vi "Make Connections (Parallel).vi"(8 "error in (no error)":errorcluster, 10 "switchActionsArray":T1 {"RelayAction" items=["CloseRelay"=21, "OpenRelay"=20]}, 11 "SLSC Switch in":refnum<class "SLSC Switch.lvclass">) -> (0 "error out":errorcluster, 3 "SLSC Switch out":refnum<class "SLSC Switch.lvclass">)   [LabVIEW 2015, in "SLSC Switch.lvclass"]
uses:
  SLSC Switch.lvclass
  slscsl/SwitchActionsArray.ctl
  slscsl/SwitchAction.ctl
  slscsl/RelayAction.ctl
  SLSC Switch.lvclass/SLSC Switch.ctl
  Relay Interface/RelayInterface.lvclass
  slscsl/slscsl.lvclass
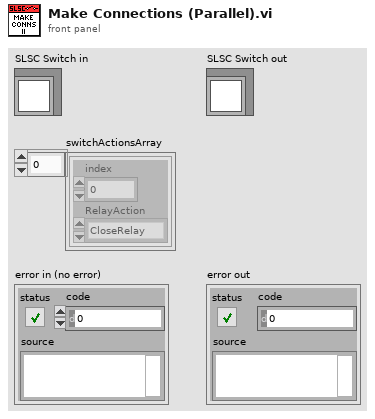
[diagram p1: front panel]
types:
  T1 = typedef "slscsl.lvclass/SwitchActionsArray.ctl" = T2[]
  T2 = typedef "slscsl.lvclass/SwitchAction.ctl" = cluster{"index":i32, "RelayAction":T3}
  T3 = typedef "slscsl.lvclass/RelayAction.ctl" = u32
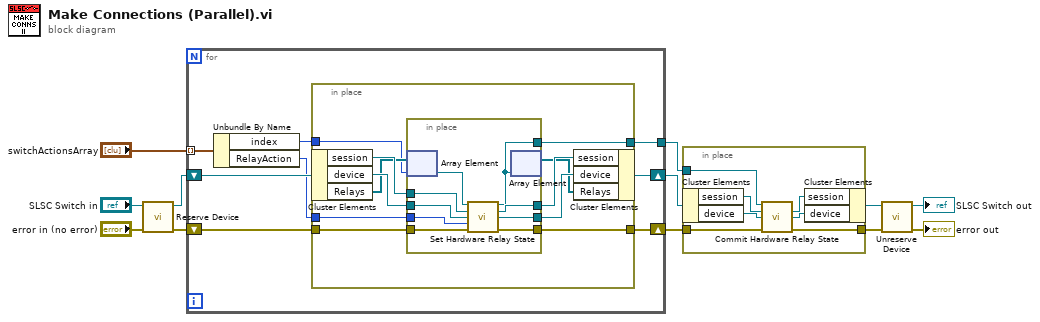
[diagram p0: block diagram]
diagram:
  n1 = call "Reserve Device.vi"("error in (no error)"="error in (no error)", "SLSC Switch in"="SLSC Switch in") -> ("error out"=w6:errorcluster, "SLSC Switch out"=w7:refnum<class "SLSC Switch.lvclass">)  [unwired: 8 in]
  n2 = for {
    tunnel: "switchActionsArray" -> [w20] mode=indexing
    shift-right: [w15] -> w5
    shift-left: w7 -> [w17]
    shift-right: [w18] -> w2
    shift-left: w6 -> [w19]
    tunnel: [w13] -> w4
    n3 = Unbundle By Name(w20) -> ("index"=w16:i32, "RelayAction"=w14:T3)
    n4 = in-place {
      in-place-border: w19 -> [w31]
      in-place-border: w14 -> [w30]
      in-place-border: [w29] -> w18
      in-place-border: w16 -> [w23]
      in-place-border: [w21] -> w13
      n5 = in-place-cluster #1(w17) -> ("session"=w28:refnum<k21>, "device"=w27:refnum<k21>, "Relays"=w24:refnum<class "RelayInterface.lvclass">[])
      n6 = in-place {
        in-place-border: w31 -> [w40]
        in-place-border: w30 -> [w39]
        in-place-border: [w34] -> w29
        in-place-border: w28 -> [w38]
        in-place-border: w27 -> [w37]
        in-place-border: [w33] -> w26
        in-place-border: [w35] -> w25
        in-place-border: [w32] -> w21
        n7 = in-place-array #2(w24, w23) -> (w36:refnum<class "RelayInterface.lvclass">)
        n8 = call-dynamic "Set Hardware Relay State.vi"("RelayInterface in"=w36, "session in"=w38, "device in"=w37, "relay action (Close Relay)"=w39, "error in (no error)"=w40) -> ("RelayInterface out"=w32:refnum<class "RelayInterface.lvclass">, "session out"=w33:refnum<k21>, "device out"=w35:refnum<k21>, "error out"=w34:errorcluster)  [unwired: 7 in]
        n9 = in-place-array #2(w32) -> (w22:refnum<class "RelayInterface.lvclass">[])  [unwired: 1 out]
      }
      n10 = in-place-cluster #1("session"=w26, "device"=w25, "Relays"=w22) -> (w15:refnum<class "SLSC Switch.lvclass">)
    }
  }
  n11 = in-place {
    in-place-border: w4 -> [w45]
    in-place-border: w2 -> [w42]
    in-place-border: [w41] -> w1
    n12 = in-place-cluster #3(w5) -> ("session"=w47:refnum<k21>, "device"=w46:refnum<k21>)
    n13 = call-dynamic "Commit Hardware Relay State.vi"("RelayInterface in"=w45, "session in"=w47, "device in"=w46, "error in (no error)"=w42) -> ("session out"=w44:refnum<k21>, "device out"=w43:refnum<k21>, "error out"=w41:errorcluster)  [unwired: 8 in, 1 out]
    n14 = in-place-cluster #3("session"=w44, "device"=w43) -> (w3:refnum<class "SLSC Switch.lvclass">)
  }
  n15 = call "Unreserve Device.vi"("error in (no error)"=w1, "SLSC Switch in"=w3) -> ("error out"=→"error out":errorcluster, "SLSC Switch out"=→"SLSC Switch out":refnum<class "SLSC Switch.lvclass">)  [unwired: 8 in]
